vi "Simple UDP - Sender.vi"() -> ()   [LabVIEW 2018]
doc: "The UDP protocol differs from TCP in that there is no error-checking with the packets of information that are sent, and thus no guarantee whatsoever that an intended recipient will actually receive a given piece of data.\n\nUDP does offer the ability to \"broadcast\" data across a network--simply specify an IP Address of all ones (255.255.255.255) to attempt to broadcast information network-wide. Keep in mind that routers and other network hardware will generally refuse to forward the broadcast beyond certain points, so the extent of the broadcast will in practice be limited."
panel:
  in  "myRIO Address":string="172.16.0.1"
  out "Message":i32
  in  "Stop":bool
  # "Überblick: Sende UDP-Messages zu myRIO. Zähler bis 60, jede Sekunde.\nDieses Simple UDP -Sender.vi läuft auf dem PC.\nAnleitung:\n1. Run dieses VI.\n2. Download Simple UDP - Receiver.vi auf myRIO(Sunderbird1), wenn nötig.\n3. IP Adress (Z.B. Zuhause: 192.168.1.15, eduroam:  139.13.73.146)"
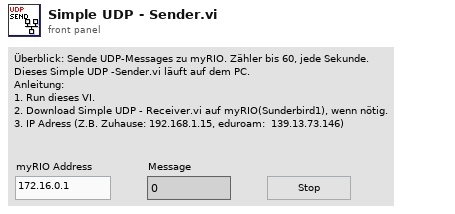
[diagram p1: front panel]
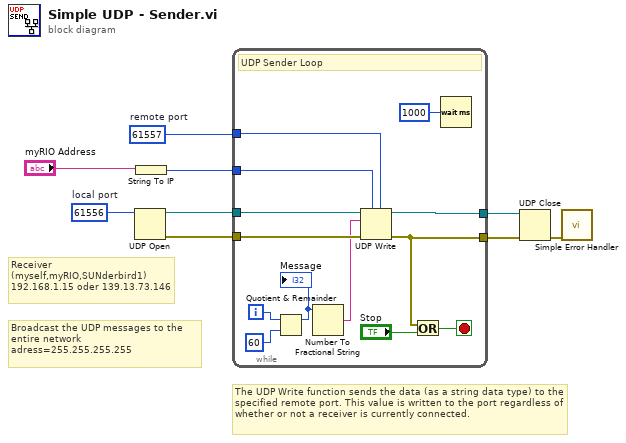
[diagram p0: block diagram]
diagram:
  w1 = u16 61557  # remote port
  w2 = u16 61556  # local port
  # "Receiver \n(myself,myRIO,SUNderbird1)\n192.168.1.15 oder 139.13.73.146"
  # "Broadcast the UDP messages to the entire network adress=255.255.255.255"
  # "The UDP Write function sends the data (as a string data type) to the specified remote port. This value is written to the port regardless of whether or not a receiver is currently connected."
  n1 = UDP Open(11:w2) -> (port=w4:refnum<k16>, 0:w3:errorcluster)  [unwired: 4 in, 1 out]
  n2 = String To IP(1:"myRIO Address") -> (0:w5:u32)
  n3 = while {
    tunnel: [w17] -> w8
    tunnel: w4 -> [w22]
    tunnel: w3 -> [w21]
    tunnel: [w18] -> w9
    tunnel: w5 -> [w16]
    tunnel: w1 -> [w13]
    i -> [w11]
    stop <- w20 stop-if-true
    # "UDP Sender Loop"
    n4 = Quotient & Remainder(x=w11, y=60 ("x")) -> (x-y*floor(x/y)=w12:i32)  [unwired: 1 out]
    "Message" <- w12
    n5 = Number To Fractional String(number=w12) -> (F-format string=w14:string)  [unwired: 3 in]
    n6 = UDP Write(address=w16, port or service name=w13, connection ID=w22, data in=w14, 8:w21) -> (error out=w17:errorcluster, 3:w18:refnum<k16>)  [unwired: 1 in]
    n7 = Or(x=w17, y="Stop") -> (x .or. y?=w20:bool)
    n8 = Wait (ms)(milliseconds to wait=u32 1000) -> ()  [unwired: 1 out]
  }
  n9 = UDP Close(connection ID=w9, 8:w8) -> (error out=w6:errorcluster)  [unwired: 1 out]
  n10 = call <vilib>:"Simple Error Handler.vi"("error in (no error)"=w6) -> ()  [unwired: 4 in, 5 out]
